vi "Reset Controls.vi"(8 "error in (no error)":errorcluster, 11 "Measurement UI in":refnum<class "Measurement UI.lvclass">) -> (0 "error out":errorcluster, 3 "Measurement UI out":refnum<class "Measurement UI.lvclass">)   [LabVIEW 2016, in "Measurement UI.lvlib" / "Measurement UI.lvclass"]
uses:
  Measurement UI.lvclass
  User Interface/UI.lvclass
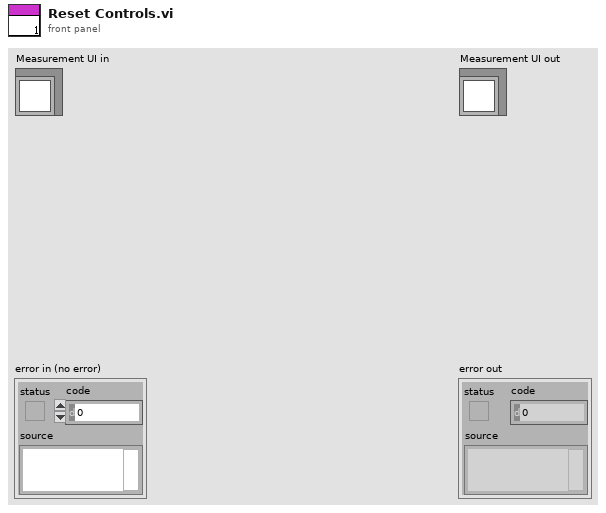
[diagram p1: front panel]
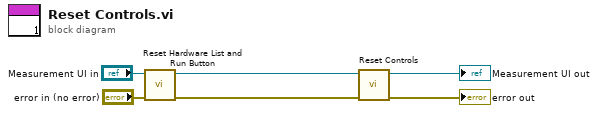
[diagram p0: block diagram]
diagram:
  n1 = call "Reset Hardware List and Run Button.vi"("error in (no error)"="error in (no error)", "Measurement UI in"="Measurement UI in") -> ("error out"=w2:errorcluster, "Measurement UI out"=w1:refnum<class "Measurement UI.lvclass">)  [unwired: 8 in]
  n2 = call-parent "Reset Controls.vi"("error in (no error)"=w2, "UI in"=w1) -> ("error out"=→"error out":errorcluster, "UI out"=→"Measurement UI out":refnum<class "Measurement UI.lvclass">)  [unwired: 8 in]
